vi "Actor Core.vi"(8 "error in":errorcluster, 11 "Timing Engine Tester in":refnum<class "Timing Engine Tester.lvclass">) -> (0 "error out":errorcluster, 3 "Actor out":refnum<class "Actor.lvclass">)   [LabVIEW 2016, in "Timing Engine Tester.lvlib" / "Timing Engine Tester.lvclass"]
doc: "(<B>Filename</B>: Actor Framework.lvlib:Actor.lvclass:Actor Core.vi)\n\nReceives messages to the actor, reacts to them, and initiates any error handling that may shut the actor down.\n\nDescendant classes may override this VI to append parallel tasks for the actor to complete while it handles messages. Overrides use the Call Parent Method node."
uses:
  Timing Engine Tester.lvclass
  C:/Program Files (x86)/National Instruments/LabVIEW 2016/vi.lib/ActorFramework/Actor/Actor.lvclass
  C:/Users/ukhornp/Documents/Work/Projects/actor_assert_api/Core/Base UI Actor/Base UI Actor/Base UI Actor.lvclass
  <vilib>/ActorFramework/Actor/Actor.lvclass
  Core/Timing Engine/Timing Engine/Timing Engine.lvclass
  Timing Engine Tester Messages/Generate Test Event Msg/Generate Test Event Msg.lvclass
  C:/Users/ukhornp/Documents/Work/Projects/actor_assert_api/Core/Timing Engine/Timing Engine Messages/Update Msg/Update Msg.lvclass
  Timing Engine Tester.lvclass/Timing Engine Tester.ctl
  Core/Timing Engine/Timing Engine/Timing Engine.lvclass/Timing Engine.ctl
  Core/Base UI Actor/Base UI Actor/Base UI Actor.lvclass/Base UI Actor.ctl
  <vilib>/ActorFramework/Actor/Actor.lvclass/Actor.ctl
  <vilib>/ActorFramework/Message Enqueuer/Message Enqueuer.lvclass/Message Enqueuer.ctl
  Timing Engine Tester Messages/Update Count Value Msg/Update Count Value Msg.lvclass/Update Count Value Msg.ctl
  <vilib>/ActorFramework/Message Enqueuer/Init from Existing Queue.vi
  <vilib>/ActorFramework/Message Enqueuer/Enqueue.vi
  Timing Engine Tester Messages/Update Count Value Msg/Update Count Value Msg.lvclass
  C:/Program Files (x86)/National Instruments/LabVIEW 2016/vi.lib/ActorFramework/Message/Message.lvclass
  <vilib>/Utility/LVClass/Get LV Class Name.vi
  <resource>/AFDebug/Generate Trace for Message.vi
  <vilib>/ActorFramework/Message Priority Queue/Priority Enqueue.vi
  <vilib>/ActorFramework/Message Enqueuer/Message Enqueuer.lvclass
  Core/Base UI Actor/Base UI Actor/Base UI Actor.lvclass
panel:
  out "Count":i32
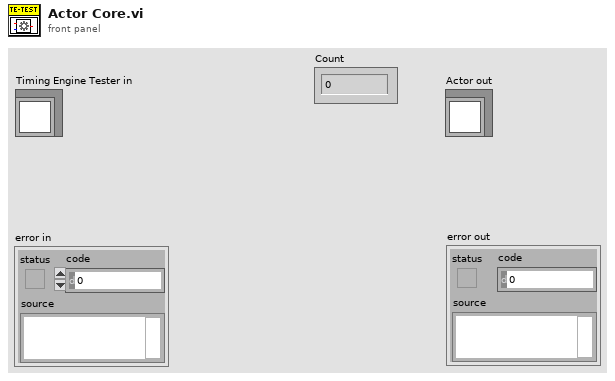
[diagram p1: front panel]
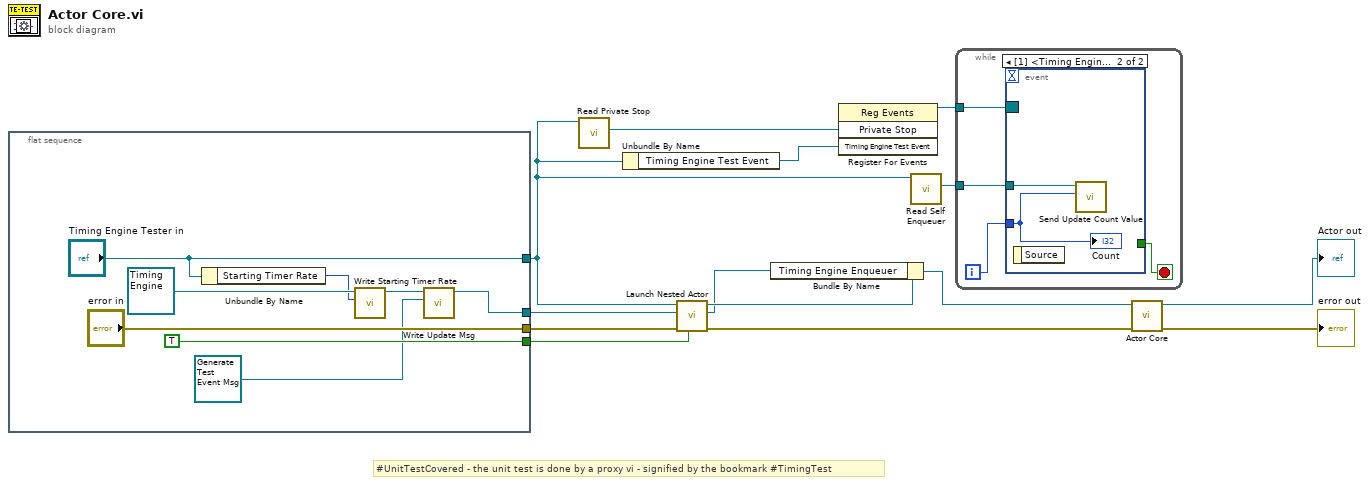
[diagram p0: block diagram]
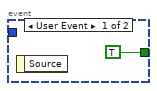
[diagram p2: hidden frame]
diagram:
  # "#UnitTestCovered - the unit test is done by a proxy vi - signified by the bookmark #TimingTest"
  n1 = flat-sequence {
    tunnel: ["error in"] -> w13
    tunnel: [TRUE ("Open Actor Core front panel? (F)")] -> w10
    tunnel: [w19] -> w9
    tunnel: ["Timing Engine Tester in"] -> w5
    frame #0 {
      n2 = Unbundle By Name("Timing Engine Tester in") -> ("Starting Timer Rate"=w15:i32)
      n3 = call "Write Starting Timer Rate.vi"("Starting Timer Rate"=w15, "Timing Engine in"=refnum<class "Timing Engine.lvclass"> refnum ("Assert API Components.lvlib:Assert Display.lvlib:Timing Engine.lvlib:Timing Engine.lvclass")) -> ("Timing Engine out"=w17:refnum<class "Timing Engine.lvclass">)  [unwired: 8 in, 1 out]
      n4 = call "Write Update Msg.vi"("Update Msg.lvclass"=refnum<class "Generate Test Event Msg.lvclass"> refnum ("Assert API Components.lvlib:Assert Display.lvlib:Timing Engine Tester.lvlib:Generate Test Event Msg.lvclass"), "Timing Engine in"=w17) -> ("Timing Engine out"=w19:refnum<class "Timing Engine.lvclass">)  [unwired: 9 in]
    }
  }
  n5 = call "Read Private Stop.vi"("Base UI Actor in"=w5) -> ("Private Stop"=w4:refnum<user-event>)  [unwired: 10 in]
  n6 = Unbundle By Name(w5) -> ("Timing Engine Test Event"=w7:refnum<user-event>)
  n7 = call <vilib>:"Launch Nested Actor.vi"("Open Actor Core front panel? (F)"=w10, "error in (no error)"=w13, "Nested Actor"=w9, "Caller Actor in"=w5) -> ("error out"=w12:errorcluster, "Nested Actor's Enqueuer"=w1:refnum<class "Message Enqueuer.lvclass">, "Caller Actor out"=w11:refnum<class "Timing Engine Tester.lvclass">)  [unwired: 5 in]
  n8 = Bundle By Name(cluster=w11, "Timing Engine Enqueuer"=w1) -> (w2:refnum<class "Timing Engine Tester.lvclass">)
  n9 = register-events(w4, w7) -> (reference out=w6:refnum<event-registration>)  [unwired: 2 in, 1 out]
  n10 = call <vilib>:"Read Self Enqueuer.vi"("Actor"=w5) -> ("Self Enqueuer"=w8:refnum<class "Message Enqueuer.lvclass">)  [unwired: 10 in]
  n11 = while {
    tunnel: w8 -> [w26]
    tunnel: w6 -> [w23]
    i -> [w24]
    stop <- w25 stop-if-true
    n12 = event shown="[1] <Timing Engine Test Event>: User Event" {
      selector: w23 -> [_ _]
      dyn-events: _ -> [_ _]
      timeout: _ -> [_ _]
      tunnel: w26 -> [_ w29]
      tunnel: [TRUE _] -> w25
      tunnel: w24 -> [_ w28]
      event User Event {
        n13 = event-data() -> ()  [unwired: 1 in, 1 out]
      }
      event User Event {
        n14 = event-data() -> ()  [unwired: 1 in, 1 out]
        n15 = call "Send Update Count Value.vi"("Count"=w28, "Message Enqueuer"=w29) -> ()  [unwired: 8 in, 2 out]
        "Count" <- w28
      }
    }
  }
  n16 = call-parent "Actor Core.vi"("error in"=w12, "Actor in"=w2) -> ("error out"=→"error out":errorcluster, "Actor out"=→"Actor out":refnum<class "Actor.lvclass">)  [unwired: 8 in]
